vi "Kinect Standardize Cropped Image.vi"(9 "Height":i32=100, 10 "Width":i32=100, 11 "Image":T1(plugin-control)) -> (2 "Image Dst Out":T1(plugin-control), 3 "Image Original Out":T1)   [LabVIEW 2011]
uses:
  <vilib>/vision/Image Controls.llb/IMAQ Image.ctl
  <vilib>/vision/NI_Vision_Development_Module.lvlib
panel:
  out "Y Axis Averages":sgl[](array[numeric]) format="%.2f"
  out "X Axis Averages":sgl[](array[numeric]) format="%.2f"
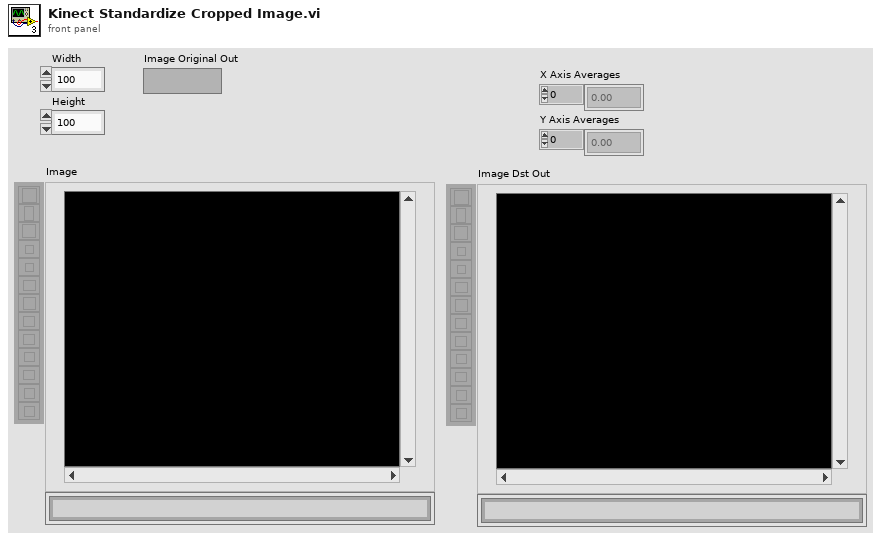
[diagram p1: front panel]
types:
  T1 = typedef "IMAQ Image.ctl" = refnum<image>
  T2 = typedef "Image Type" = u32
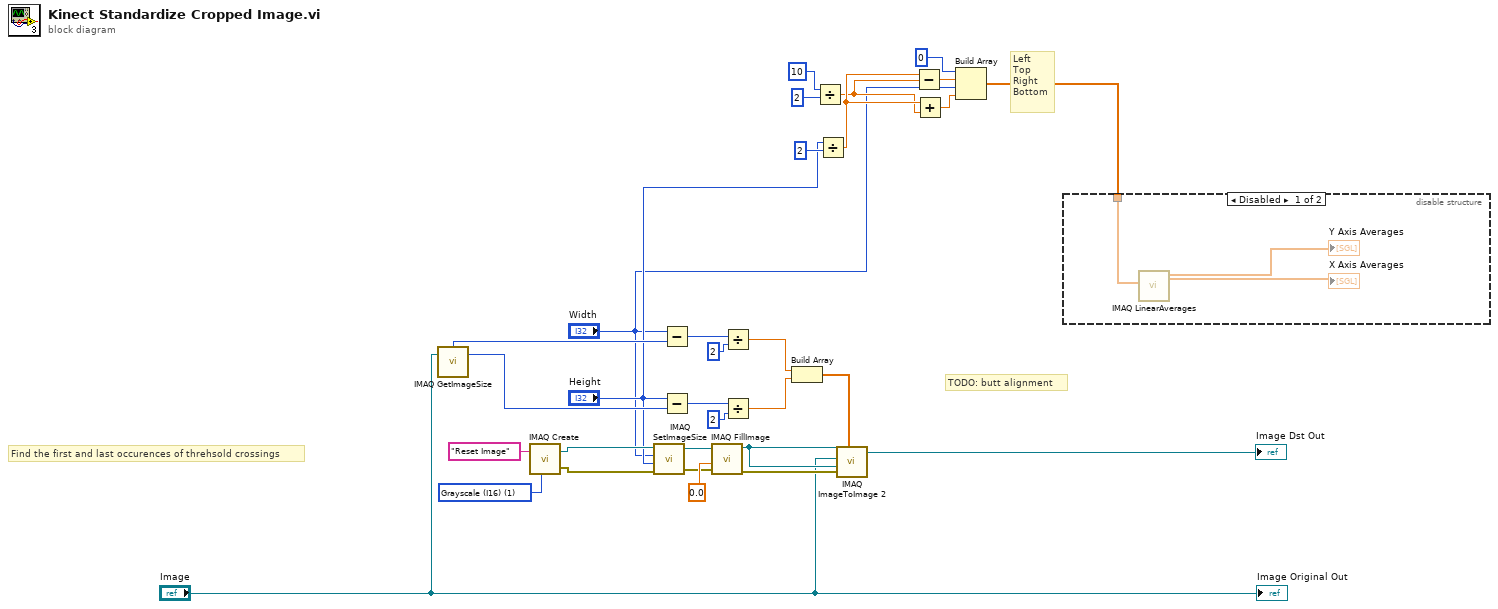
[diagram p0: block diagram]
diagram:
  w28 = T2 1 items=["Grayscale (U8)", "Grayscale (I16)", "Grayscale (SGL)", "Complex (CSG)", "RGB (U32)", "HSL (U32)", "RGB (U64)", "Grayscale (U16)"] ("Image Type")
  # "Left\nTop\nRight\nBottom"
  # "Find the first and last occurences of threhsold crossings"
  # "TODO: butt alignment"
  n1 = call "IMAQ GetImageSize"("Image"="Image") -> ("Y Resolution"=w21:i32, "X Resolution"=w22:i32)  [unwired: 3 in, 1 out]
  n2 = call "IMAQ Create"("Image Name"="Reset Image", "Image Type"=w28) -> ("New Image"=w19:T1, "error out"=w18:errorcluster)  [unwired: 3 in]
  n3 = call "IMAQ SetImageSize"("error in (no error)"=w18, "Y Resolution"="Height", "X Resolution"="Width", "Image"=w19) -> ("error out"=w15:errorcluster, "Image Out"=w17:T1)  [unwired: 1 in]
  n4 = Subtract(x="Width", y=w22) -> (x-y=w26:i32)
  n5 = Subtract(x="Height", y=w21) -> (x-y=w27:i32)
  n6 = call "IMAQ FillImage"("error in (no error)"=w15, "Pixel Value (U8, U16, I16, Float)"=sgl 0.0, "Image"=w17) -> ("error out"=w14:errorcluster, "Image Out"=w13:T1)  [unwired: 7 in]
  n7 = Divide(x=w26, y=2) -> (x/y=w25:dbl)
  n8 = Divide(x=w27, y=2) -> (x/y=w24:dbl)
  n9 = Build Array(w25, w24) -> (w23:dbl[])
  n10 = Divide(x=10 ("Width of Band to \nCalculate Average Contour"), y=2) -> (x/y=w4:dbl)
  n11 = Divide(x="Height", y=2) -> (x/y=w5:dbl)
  n12 = call "IMAQ ImageToImage 2"("Offset Left/Top"=w23, "error in (no error)"=w14, "Image Dst"=w13, "Image Src (Small)"="Image", "Image Src (Large)"=w13) -> ("Image Dst Out"=→"Image Dst Out":T1)  [unwired: 5 in, 1 out]
  n13 = Subtract(x=w5, y=w4) -> (x-y=w7:dbl)
  n14 = Add(x=w5, y=w4) -> (x+y=w6:dbl)
  n15 = Build Array(0 ("element"), w7, "Width", w6) -> (w3:dbl[])
  n16 = disable-structure shown="Disabled" {
    disable-tunnel: w3 -> [w34 _]
    frame Disabled {
      n17 = call "IMAQ LinearAverages"("Optional Rectangle"=w34) -> ("Y Axis Averages"=→"Y Axis Averages":sgl[], "X Axis Averages"=→"X Axis Averages":sgl[])  [unwired: 6 in, 3 out]
    }
    frame Enabled {
    }
  }
  "Image Original Out" <- "Image"
